vi "Go To Destroy.vi"(7 "Sender":refnum<class "Sender.lvclass">, 11 "Go To Destroy in":refnum<class "Go To Destroy.lvclass">) -> (0 "Error out":errorcluster, 3 "Go To Destroy out":refnum<class "Go To Destroy.lvclass">)   [LabVIEW 2020, in "jettl.lvlib" / "Go To Destroy Msg.lvlib" / "Go To Destroy.lvclass"]
uses:
  Go To Destroy.lvclass
  Sender/Sender/Sender.lvclass
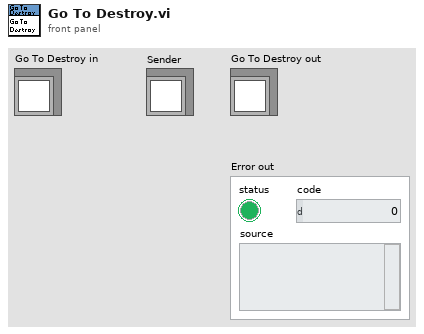
[diagram p1: front panel]
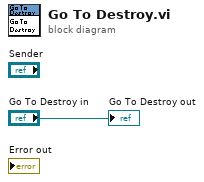
[diagram p0: block diagram]
diagram:
  "Go To Destroy out" <- "Go To Destroy in"
